vi "ID Parser.vi"(8 "error in (no error)":errorcluster, 10 "ID":string, 11 "Control System Object in":refnum<class "Control System Object.lvclass">) -> (0 "error out":errorcluster, 3 "Control System Object out":refnum<class "Control System Object.lvclass">)   [LabVIEW 2014, in "Control System Object.lvlib" / "Control System Object.lvclass"]
uses:
  Control System Object.lvclass
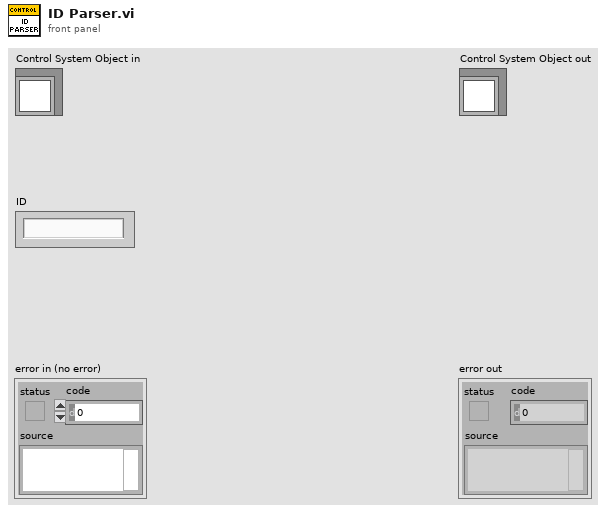
[diagram p1: front panel]
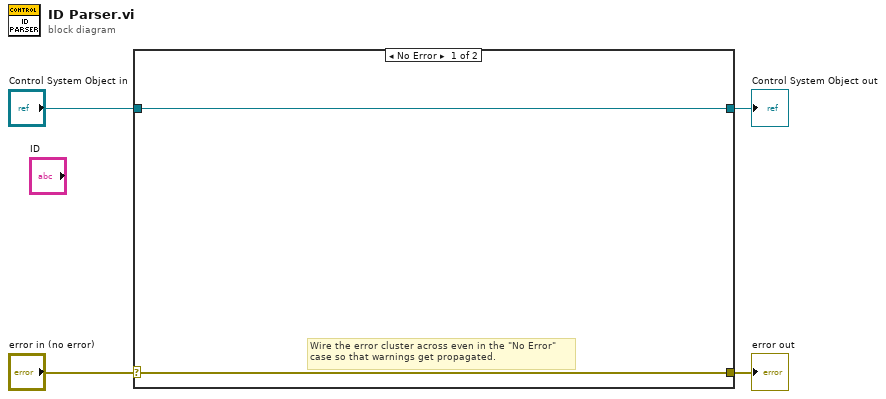
[diagram p0: block diagram]
diagram:
  n1 = case shown="No Error" "error in (no error)" {
    selector: "error in (no error)" -> [w5 w8]
    tunnel: [w5 w8] -> w3
    tunnel: [w6 w7] -> w1
    tunnel: "Control System Object in" -> [w6 w7]
    frame No Error {
      # "Wire the error cluster across even in the \"No Error\"\ncase so that warnings get propagated."
    }
    frame Error {
    }
  }
  "error out" <- w3
  "Control System Object out" <- w1
